vi "Read-SRC-all-varid.vi"(11 "entrée erreur":errorcluster caption="err (in)") -> (4 "tb-ent":string[](array[string]), 6 "tb-2D_src":string[][](array[string]), 10 "1D_src":T1[](array[typedef]), 15 "error out":errorcluster caption="err (out)")   [LabVIEW 2010, in "lv_04.lvlib"]
uses:
  lv_04.lvlib
  commandes/cSTA_varid.ctl
  commandes/c_TDMS_ch_variable.ctl
  commandes/c_TDMS_ch_donnees.ctl
  commandes/c0-var-n.ctl
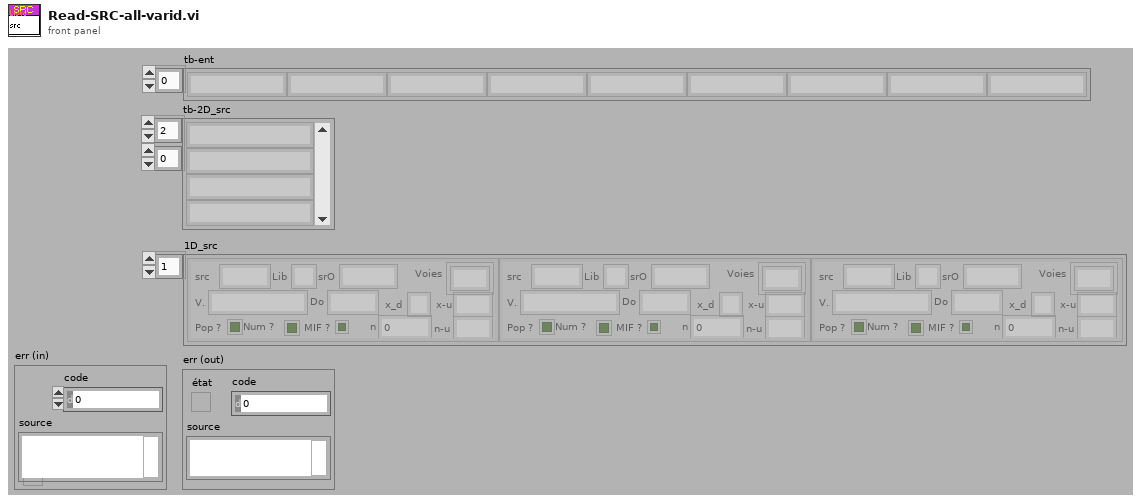
[diagram p1: front panel]
types:
  T1 = typedef "lv_04.lvlib/cSTA_varid.ctl" = cluster{"src":string, "Lib":string, "srO":string, "V.":T2, "Voies":string[], "Do":T3, "n":T4, "Num ?":bool, "Pop ?":bool, "x_d":string, "x-u":string, "n-u":string, "MIF ?":bool}
  T2 = typedef "lv_04.lvlib/c_TDMS_ch_variable.ctl" = string
  T3 = typedef "lv_04.lvlib/c_TDMS_ch_donnees.ctl" = string
  T4 = typedef "lv_04.lvlib/c0-var-n.ctl" = i32
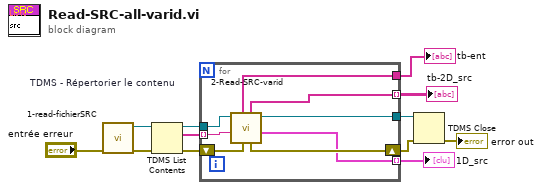
[diagram p0: block diagram]
diagram:
  n1 = call "1-read-fichierSRC.vi"("err in"="entrée erreur") -> ("err out"=w11:errorcluster, "tdms file out"=w10:refnum<k34>)  [unwired: 4 in, 1 out]
  n2 = TDMS List Contents "TDMS - Répertorier le contenu"(4:w11, 7:w10) -> (0:w6:errorcluster, 2:w8:string[], 3:w7:refnum<k34>)  [unwired: 1 in, 1 out]
  n3 = for {
    tunnel: w8 -> [w15] mode=indexing
    tunnel: w7 -> [w20]
    shift-right: [w18] -> w4
    shift-left: w6 -> [w19]
    tunnel: [w16] -> w5
    tunnel: [w17] -> w3 mode=indexing
    tunnel: [w14] -> w2
    tunnel: [w13] -> w1 mode=indexing
    n4 = call "2-Read-SRC-varid.vi"("err in"=w19, "code src"=w15, "tdms in"=w20) -> ("varid"=w13:T1, "tdms out"=w16:refnum<k34>, "error out"=w18:errorcluster, "txt_desc_TDMS"=w17:string[], "ent_desc_TDMS"=w14:string[])  [unwired: 4 in]
  }
  "tb-2D_src" <- w3
  "tb-ent" <- w2
  "1D_src" <- w1
  n5 = TDMS Close(8:w4, 11:w5) -> (0:→"error out":errorcluster)  [unwired: 1 out]
